vi "test11-TestArgumentInfoOfTriggeredState_Status.vi"(8 "error in (no error)":errorcluster, 11 "TestCase in":refnum<class "testcase-CSMStatusStateRegisterUnregister.lvclass">) -> (0 "error out":errorcluster, 3 "TestCase out":refnum<class "testcase-CSMStatusStateRegisterUnregister.lvclass">)   [LabVIEW 2017, in "testcase-CSMStatusStateRegisterUnregister.lvclass"]
uses:
  testcase-CSMStatusStateRegisterUnregister.lvclass
  src/user.lib/_NEVSTOP/Communicable State Machine(CSM)/_Support/Typedef/_CSM_List Module Scope.ctl
  bc269a46-fbd8-4fbd-ac76-06990d02385a.vi
  8d37a2f4-20d8-4102-818c-5a8acec6f80e.vi
  src/user.lib/_NEVSTOP/Communicable State Machine(CSM)/AdvanceAPI/CSM - Get Module Attribute.vi
  <vilib>/addons/_JKI Toolkits/VI Tester/TestCase.llb/TestCase.lvclass
  src/user.lib/_NEVSTOP/Communicable State Machine(CSM)/Communicable State Machine.lvlib
  C:/Program Files (x86)/National Instruments/LabVIEW 2017/vi.lib/addons/_JKI Toolkits/VI Tester/TestCase.llb/TestCase.lvclass
panel:
  out "LoopCount":i32
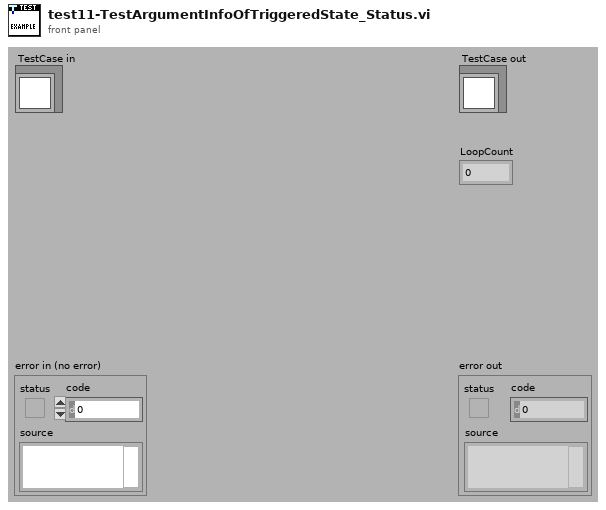
[diagram p1: front panel]
types:
  T1 = typedef "Communicable State Machine.lvlib/_CSM_List Module Scope.ctl" = enum16{"Normal", "System Only", "All"}
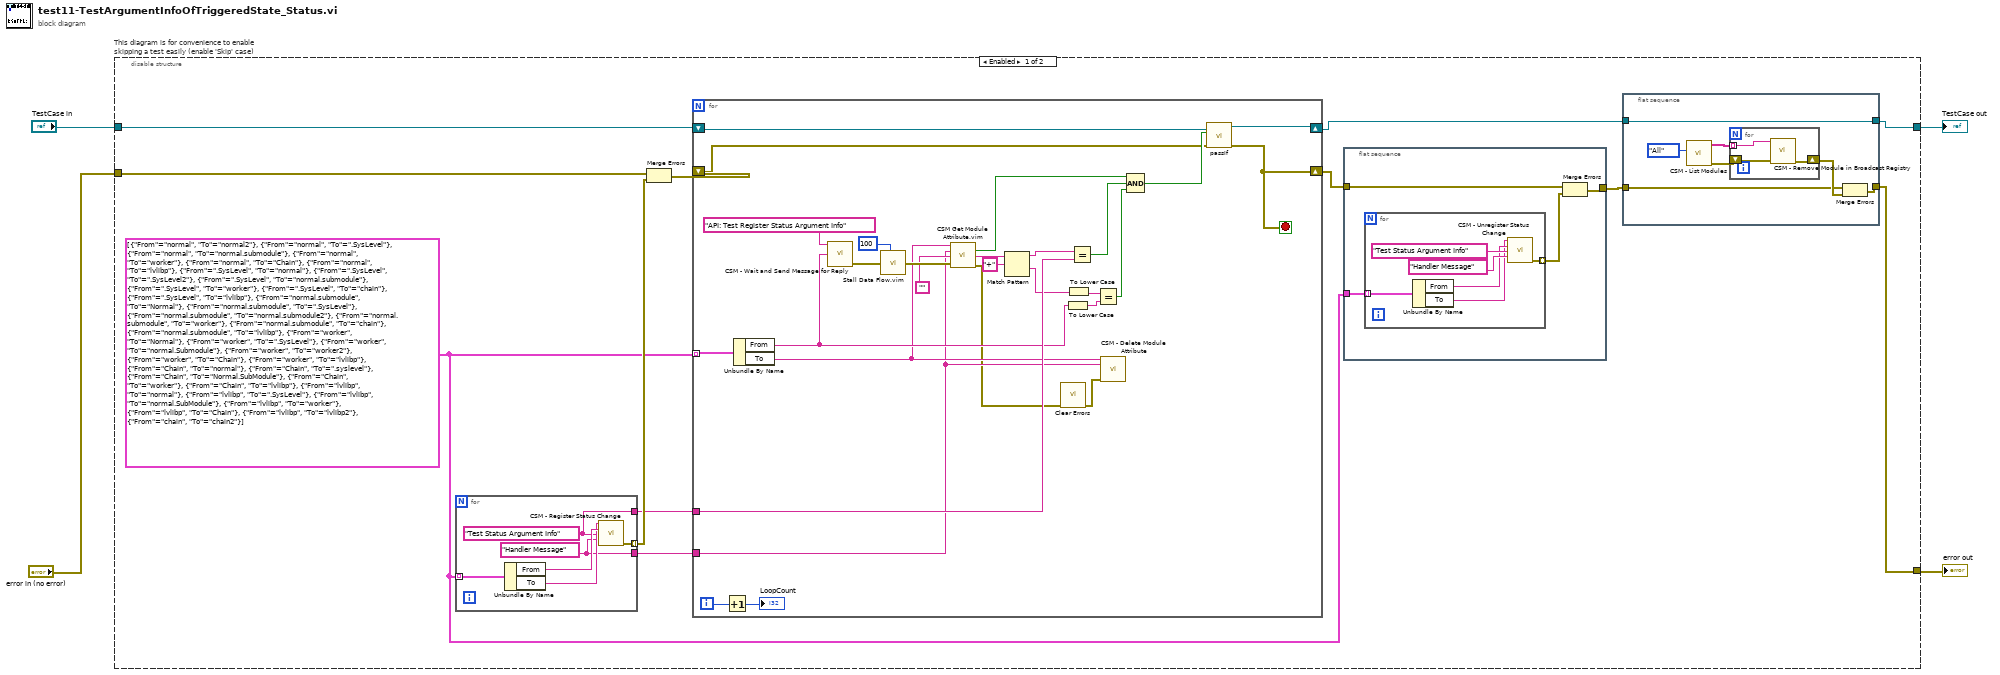
[diagram p0: block diagram]
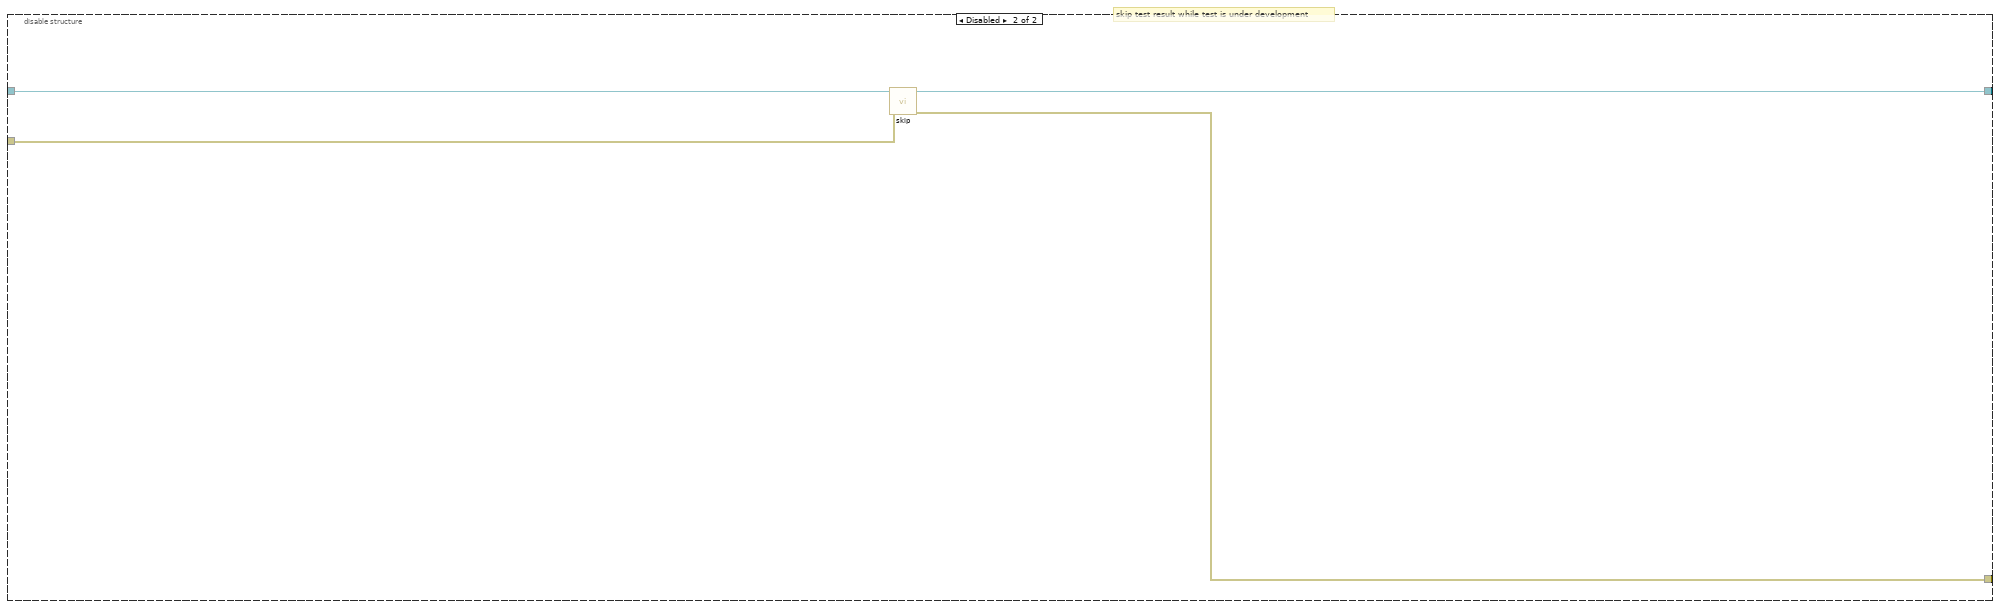
[diagram p2: hidden frame]
diagram:
  n1 = disable-structure "This diagram is for convenience to enable skipping a test easily (enable 'Skip' case)" shown="Enabled" {
    disable-tunnel: "TestCase in" -> [w16 w74]
    disable-tunnel: [w6 w72] -> w2
    disable-tunnel: [w9 w73] -> w1
    disable-tunnel: "error in (no error)" -> [w15 w71]
    frame Enabled {
      w12 = cluster{"From":string, "To":string}[] [{"From"="normal", "To"="normal2"}, {"From"="normal", "To"=".SysLevel"}, {"From"="normal", "To"="normal.submodule"}, {"From"="normal", "To"="worker"}, {"From"="normal", "To"="Chain"}, {"From"="normal", "To"="lvlibp"}, {"From"=".SysLevel", "To"="normal"}, {"From"=".SysLevel", "To"=".SysLevel2"}, {"From"=".SysLevel", "To"="normal.submodule"}, {"From"=".SysLevel", "To"="worker"}, {"From"=".SysLevel", "To"="chain"}, {"From"=".SysLevel", "To"="lvlibp"}, {"From"="normal.submodule", "To"="Normal"}, {"From"="normal.submodule", "To"=".SysLevel"}, {"From"="normal.submodule", "To"="normal.submodule2"}, {"From"="normal.submodule", "To"="worker"}, {"From"="normal.submodule", "To"="chain"}, {"From"="normal.submodule", "To"="lvlibp"}, {"From"="worker", "To"="Normal"}, {"From"="worker", "To"=".SysLevel"}, {"From"="worker", "To"="normal.Submodule"}, {"From"="worker", "To"="worker2"}, {"From"="worker", "To"="Chain"}, {"From"="worker", "To"="lvlibp"}, {"From"="Chain", "To"="normal"}, {"From"="Chain", "To"=".syslevel"}, {"From"="Chain", "To"="Normal.SubModule"}, {"From"="Chain", "To"="worker"}, {"From"="Chain", "To"="lvlibp"}, {"From"="lvlibp", "To"="normal"}, {"From"="lvlibp", "To"=".SysLevel"}, {"From"="lvlibp", "To"="normal.SubModule"}, {"From"="lvlibp", "To"="worker"}, {"From"="lvlibp", "To"="Chain"}, {"From"="lvlibp", "To"="lvlibp2"}, {"From"="chain", "To"="chain2"}]
      n2 = for {
        tunnel: w12 -> [w32] mode=indexing
        tunnel: [w29] -> w13 mode=indexing
        tunnel: [w28] -> w8
        tunnel: [w27] -> w5
        w27 = "Handler Message" ("Response Message (If \"\", Same as Source Message)")
        w28 = "Test Status Argument Info" ("Status")
        n3 = Unbundle By Name(w32) -> ("From"=w31:string, "To"=w30:string)
        n4 = call "CSM - Register Status Change.vi"("CSM Name"=w30, "Source CSM Name (* as Default)"=w31, "Status"=w28, "Response Message (If \"\", Same as Source Message)"=w27) -> ("error out"=w29:errorcluster)  [unwired: 10 in, 1 out]
      }
      n5 = Merge Errors(w15, w13) -> (w14:errorcluster)
      n6 = for {
        tunnel: w12 -> [w69] mode=indexing
        shift-right: [w52] -> w7
        shift-left: w16 -> [w53]
        shift-right: [w49] -> w11
        shift-left: w14 -> [w50]
        tunnel: w8 -> [w60]
        tunnel: w5 -> [w47]
        i -> [w44]
        stop <- w49 stop-if-true
        n7 = Increment(x=w44) -> (x+1=→"LoopCount":i32)
        n8 = Unbundle By Name(w69) -> ("From"=w58:string, "To"=w48:string)
        n9 = call "CSM - Wait and Send Message for Reply.vi"("State"="API: Test Register Status Argument Info", "Target Module"=w58) -> ("error out"=w68:errorcluster)  [unwired: 11 in, 2 out]
        n10 = call "Stall Data Flow.vim"("value in"=w68, "milliseconds to wait"=u32 100) -> ("value out"=w66:errorcluster)  [unwired: 1 out]
        n11 = call "CSM Get Module Attribute.vim"("CSM Name"=w48, "Attribute"=w47, "Default Value (Empty Variant)"="", "Error In"=w66) -> ("Found"=w64:bool, "Value"=w63:string, "error out"=w46:errorcluster)  [unwired: 7 in, 2 out]
        n12 = Match Pattern(string=w63, regular expression="+") -> (before substring=w61:string, after substring=w59:string)  [unwired: 1 in, 2 out]
        n13 = call <vilib>:"Clear Errors.vi"("error in (no error)"=w46) -> ("error out"=w45:errorcluster)  [unwired: 5 in, 1 out]
        n14 = To Lower Case(string=w58) -> (all lower case string=w56:string)
        n15 = To Lower Case(string=w59) -> (all lower case string=w57:string)
        n16 = Equal?(x=w61, y=w60) -> (x = y?=w55:bool)
        n17 = Equal?(x=w57, y=w56) -> (x = y?=w54:bool)
        n18 = call "CSM - Delete Module Attribute.vi"("CSM Name"=w48, "Attribute"=w47, "Error In"=w45) -> ()  [unwired: 9 in, 4 out]
        n19 = Compound Arithmetic op=AND(w64, w55, w54) -> (w51:bool)
        n20 = call-dynamic "passIf.vi"("error in (no error)"=w50, "pass"=w51, "TestCase in"=w53) -> ("error out"=w49:errorcluster, "TestCase out"=w52:refnum<class "testcase-CSMStatusStateRegisterUnregister.lvclass">)  [unwired: 7 in]
      }
      n21 = flat-sequence {
        tunnel: w12 -> [w17]
        tunnel: w11 -> [w20]
        tunnel: [w19] -> w10
        frame #0 {
          n22 = for {
            tunnel: w17 -> [w21] mode=indexing
            tunnel: [w22] -> w18 mode=indexing
            n23 = Unbundle By Name(w21) -> ("From"=w24:string, "To"=w23:string)
            n24 = call "CSM - Unregister Status Change.vi"("CSM Name"=w23, "Source CSM Name (* as Default)"=w24, "Status"="Test Status Argument Info", "Response Message (\"*\" as Default)"="Handler Message" ("Response Message (If \"\", Same as Source Message)")) -> ("error out"=w22:errorcluster)  [unwired: 10 in, 1 out]
          }
          n25 = Merge Errors(w20, w18) -> (w19:errorcluster)
        }
      }
      n26 = flat-sequence {
        tunnel: w10 -> [w35]
        tunnel: [w34] -> w9
        tunnel: [w33] -> w6
        tunnel: w7 -> [w33]
        frame #0 {
          n27 = call "CSM - List Modules.vi"("Scope (Normal)"=_CSM_List_Module_Scope."All") -> ("error out"=w37:errorcluster, "Module Names"=w38:string[])  [unwired: 9 in]
          n28 = for {
            tunnel: w38 -> [w42] mode=indexing
            shift-right: [w40] -> w39
            shift-left: w37 -> [w41]
            n29 = call "CSM - Remove Module in Broadcast Registry.vi"("CSM Name"=w42, "Error In"=w41) -> ("error out"=w40:errorcluster)  [unwired: 12 in, 1 out]
          }
          n30 = Merge Errors(w35, w39) -> (w34:errorcluster)
        }
      }
    }
    frame Disabled {
      # "skip test result while test is under development"
      n31 = call <vilib>:"skip.vi"("error in (no error)"=w71, "TestCase in"=w74) -> ("error out"=w73:errorcluster, "TestCase out"=w72:refnum<class "testcase-CSMStatusStateRegisterUnregister.lvclass">)  [unwired: 8 in]
    }
  }
  "error out" <- w1
  "TestCase out" <- w2
